vi "Loop_ACT.vi"() -> ()   [LabVIEW 2017, in "Arm.lvlib"]
uses:
  Arm.lvlib
  _SHARE ALL/Global Share All/Global_STOP.vi
  Global_ACT Write_Data Out.vi
  Global_SM Write_Data Out.vi
  System Drivers/Phoenix-LabVIEW/Motor Controller/Controls/CTRE_Phoenix_MotorControl_NeutralMode.ctl
  System Drivers/Phoenix-LabVIEW/Motor Controller/Controls/CTRE_Phoenix_MotorControl_ControlMode.ctl
  CLUSTER_ElbowCMD.ctl
panel:
  out "Output Data":dbl
  out "Input Data":dbl
  out "Cycle Time (S)":dbl format="%.3g"
  in  "Target Time(ms)":u32=50
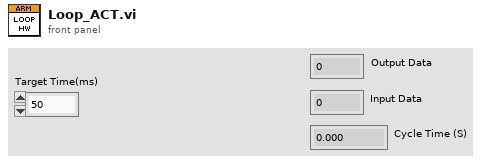
[diagram p1: front panel]
types:
  T1 = typedef "CTRE_Phoenix_MotorControl_ControlMode.ctl" = u16
  T2 = typedef "Arm.lvlib/CLUSTER_ElbowCMD.ctl" = cluster{"Talon Mode":T1}
  T3 = typedef "CTRE_Phoenix_MotorControl_NeutralMode.ctl" = enum8{"EEPROMSetting", "Override to Coast", "Override to Brake"}
  T4 = typedef "WPI_MotorControlDeviceRef.ctl" = cluster{"DeviceStatus":errorcluster, "Type":T5, "PWM":cluster{"PWM Channel":T6, "DeadBand":T7}, "CAN":cluster{"Device Number":u8, "SetOutput VI Ref":variant, "GetOutput VI Ref":variant, "Enable VI Ref":variant, "Disable VI Ref":variant, "Data":variant}, "Invert":bool, "DIO PWM":cluster{"PWM \"Enable\" Channel":T6, "DIOChannel":T8, "PWM Rate":dbl}}
  T5 = typedef "WPI_MotorControlType.ctl" = enum16{"PWM", "CAN", "DIO PWM"}
  T6 = typedef "FPGA_DIOPWMChannel.ctl" = enum8{"PWM 0", "PWM 1", "PWM 2", "PWM 3", "PWM 4", "PWM 5", "PWM 6", "PWM 7", "PWM 8", "PWM 9", "PWM MXP 0", "PWM MXP 1", "PWM MXP 2", "PWM MXP 3", "PWM MXP 4", "PWM MXP 5", "PWM MXP 6", "PWM MXP 7", "PWM MXP 8", "PWM MXP 9", "Invalid"}
  T7 = typedef "WPI_PWMDeadband.ctl" = cluster{"Name":string, "maxPositivePwm":i32, "minPositivePwm":i32, "centerPwm":i32, "maxNegativePwm":i32, "minNegativePwm":i32, "angularRange":u16}
  T8 = typedef "FPGA_DIOChannel.ctl" = enum8{"DIO 0", "DIO 1", "DIO 2", "DIO 3", "DIO 4", "DIO 5", "DIO 6", "DIO 7", "DIO 8", "DIO 9", "DIO MXP 0", "DIO MXP 1", "DIO MXP 2", "DIO MXP 3", "DIO MXP 4", "DIO MXP 5", "DIO MXP 6", "DIO MXP 7", "DIO MXP 8", "DIO MXP 9", "DIO MXP 10", "DIO MXP 11", "DIO MXP 12", "DIO MXP 13", "DIO MXP 14", "DIO MXP 15", "SPI Port CS1", "SPI Port CS2", "SPI Port CS3", "SPI Port MISO", "SPI Port MOSI", "Invalid"}
  T9 = cluster{"PhoenixMotorControlDevRef":T4, " Actuator Output":dbl, "Actuator Input":dbl, "Target Time(ms)":u32, "Current Time":timestamp, "Previous Time":timestamp, "Cycle Time (S)":dbl}
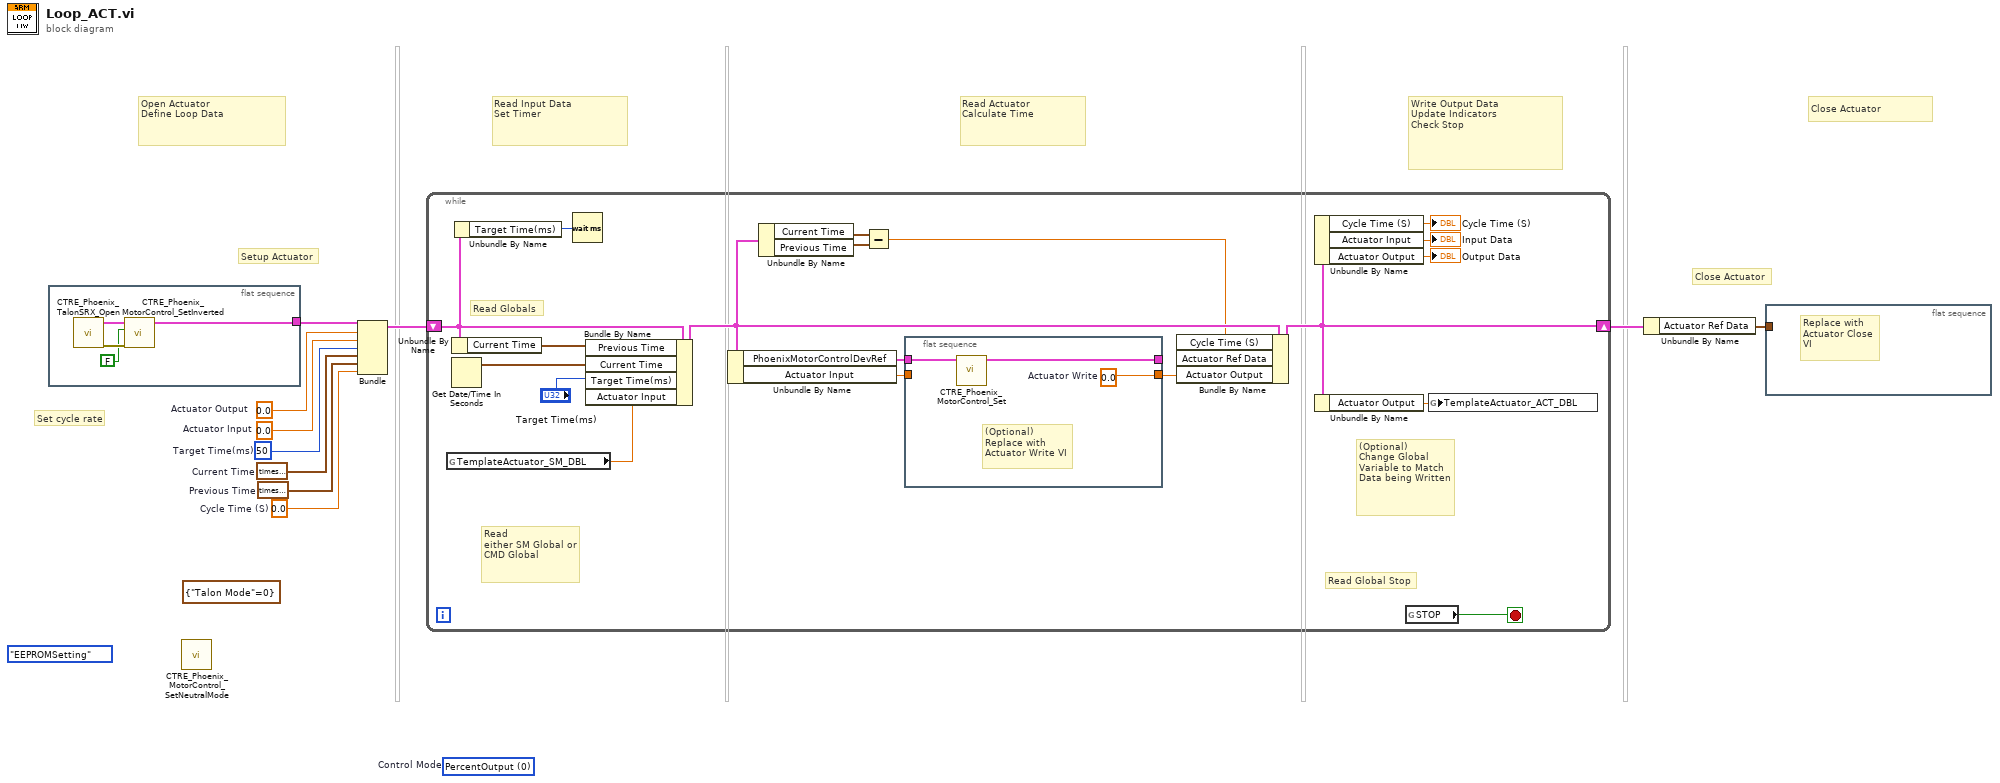
[diagram p0: block diagram]
diagram:
  (unwired) T1 0 items=["PercentOutput"=0, "Position"=1, "Velocity"=2, "Current"=3, "Follower"=5, "MotionProfile"=6, "MotionMagic"=7, "MotionMagicArc"=8, "MotionProfileArc"=10, "Disabled"=15]  # Control Mode
  (unwired) T2 {"Talon Mode"=0} ("Elbow Input")
  (unwired) CTRE_Phoenix_MotorControl_NeutralMode."EEPROMSetting" ("Motor Control Neutral Mode")
  w2 = 0.0  # Cycle Time (S)
  w10 = timestamp(0 s since 1904-01-01)  # Previous Time
  w9 = timestamp(0 s since 1904-01-01)  # Current Time
  w8 = u32 50  # Target Time(ms)
  w6 = 0.0  # Actuator Input
  w4 = 0.0  # Actuator Output
  # "Close Actuator"
  # "Write Output Data\nUpdate Indicators\nCheck Stop"
  # "Read Actuator\nCalculate Time"
  # "Read Input Data\nSet Timer"
  # "Open Actuator\nDefine Loop Data"
  # "Set cycle rate"
  # "Close Actuator"
  # "Setup Actuator"
  n1 = flat-sequence {
    tunnel: [w11] -> w1
    frame #0 {
      n2 = call "CTRE_Phoenix_TalonSRX_Open.vi"() -> ("error out"=w14:errorcluster, "CAN Talon SRX Ref"=w13:T4)  [unwired: 10 in]
      n3 = call "CTRE_Phoenix_MotorControl_SetInverted.vi"("error in (no error)"=w14, "Invert?"=FALSE, "PhoenixMotorControlDevRef"=w13) -> ("PhoenixMotorControlDevRef"=w11:T4)  [unwired: 7 in, 1 out]
    }
  }
  n4 = call "CTRE_Phoenix_MotorControl_SetNeutralMode.vi"() -> ()  [unwired: 10 in, 2 out]
  n5 = Bundle("PhoenixMotorControlDevRef"=w1, "Actuator Output"=w4, "Actuator Input"=w6, "Target Time(ms)"=w8, "Current Time"=w9, "Previous Time"=w10, "Cycle Time (S)"=w2) -> (w5:T9)  [unwired: 1 in]
  n6 = while {
    shift-right: [w21] -> w3
    shift-left: w5 -> [w23]
    stop <- w33 stop-if-true
    # "(Optional)\nChange Global\nVariable to Match\nData being Written"
    # "Read\neither SM Global or CMD Global"
    # "Read Globals"
    # "Read Global Stop"
    n7 = global read "Global_SM Write_Data Out.vi" "TemplateActuator_SM_DBL"() -> (w15:dbl)
    n8 = Unbundle By Name(w23) -> ("Current Time"=w28:timestamp)
    n9 = Get Date/Time In Seconds() -> (seconds since 1Jan1904=w29:timestamp)
    n10 = Unbundle By Name(w23) -> ("Target Time(ms)"=w22:u32)
    n11 = Wait (ms)(milliseconds to wait=w22) -> ()  [unwired: 1 out]
    n12 = Bundle By Name(cluster=w23, "Previous Time"=w28, "Current Time"=w29, "Target Time(ms)"="Target Time(ms)", "Actuator Input"=w15) -> (w24:T9)
    n13 = Unbundle By Name(w24) -> ("PhoenixMotorControlDevRef"=w32:T4, "Actuator Input"=w31:dbl)
    n14 = Unbundle By Name(w24) -> ("Current Time"=w27:timestamp, "Previous Time"=w26:timestamp)
    n15 = Subtract(x=w27, y=w26) -> (x-y=w17:dbl)
    n16 = flat-sequence {
      tunnel: w32 -> [w35]
      tunnel: [w34] -> _
      tunnel: [w36] -> w30
      tunnel: w31 -> [_]
      frame #0 {
        w36 = 0.0  # Actuator Write
        # "(Optional)\nReplace with\nActuator Write VI"
        n17 = call "CTRE_Phoenix_MotorControl_Set.vi"("PhoenixMotorControlDevRef"=w35) -> ("PhoenixMotorControlDevRef"=w34:T4)  [unwired: 9 in, 1 out]
      }
    }
    n18 = Bundle By Name(cluster=w24, "Cycle Time (S)"=w17, "Actuator Output"=w30) -> (w21:T9)  [unwired: 1 in]
    n19 = Unbundle By Name(w21) -> ("Cycle Time (S)"=→"Cycle Time (S)":dbl, "Actuator Input"=→"Input Data":dbl, "Actuator Output"=→"Output Data":dbl)
    n20 = Unbundle By Name(w21) -> ("Actuator Output"=w16:dbl)
    n21 = global read "Global_STOP.vi" "STOP"() -> (w33:bool)
    n22 = global write "Global_ACT Write_Data Out.vi" "TemplateActuator_ACT_DBL"(w16) -> ()
  }
  n23 = Unbundle By Name(w3) -> ("Actuator Ref Data"=w7:cluster{i32})
  n24 = flat-sequence {
    tunnel: w7 -> [_]
    frame #0 {
      # "Replace with \nActuator Close\nVI"
    }
  }
